vi "ElmoInterface.vi"(0 "Elmo State Cluster In":T1, 1 "Axis No.":u32, 5 "IO Signals":T2, 7 "Enable":bool, 9 "Clear faults":bool, 11 "Home":bool) -> (4 "Elmo State Cluster Out":T1, 6 "State String":string, 15 "Control word":u16)   [LabVIEW 2018]
uses:
  Clusters/IOSignals.ctl
  Clusters/ElmoState.ctl
  Clusters/SimulationConstants.ctl
  <vilib>/functionblocks/Edge Detection/Edge Detect/Edge Detect.vi
  <vilib>/functionblocks/FB Core/FB Core.xnode
  <vilib>/functionblocks/NI_FunctionBlock Libraries.lvlib
panel:
  out "Warning (Bit7)":bool
  out "Switch on disabled (Bit6)":bool
  out "Fault (Bit3)":bool
  out "Operation Enabled (Bit2)":bool
  out "Switched On (Bit1)":bool
  out "Ready to Switch On (Bit0)":bool
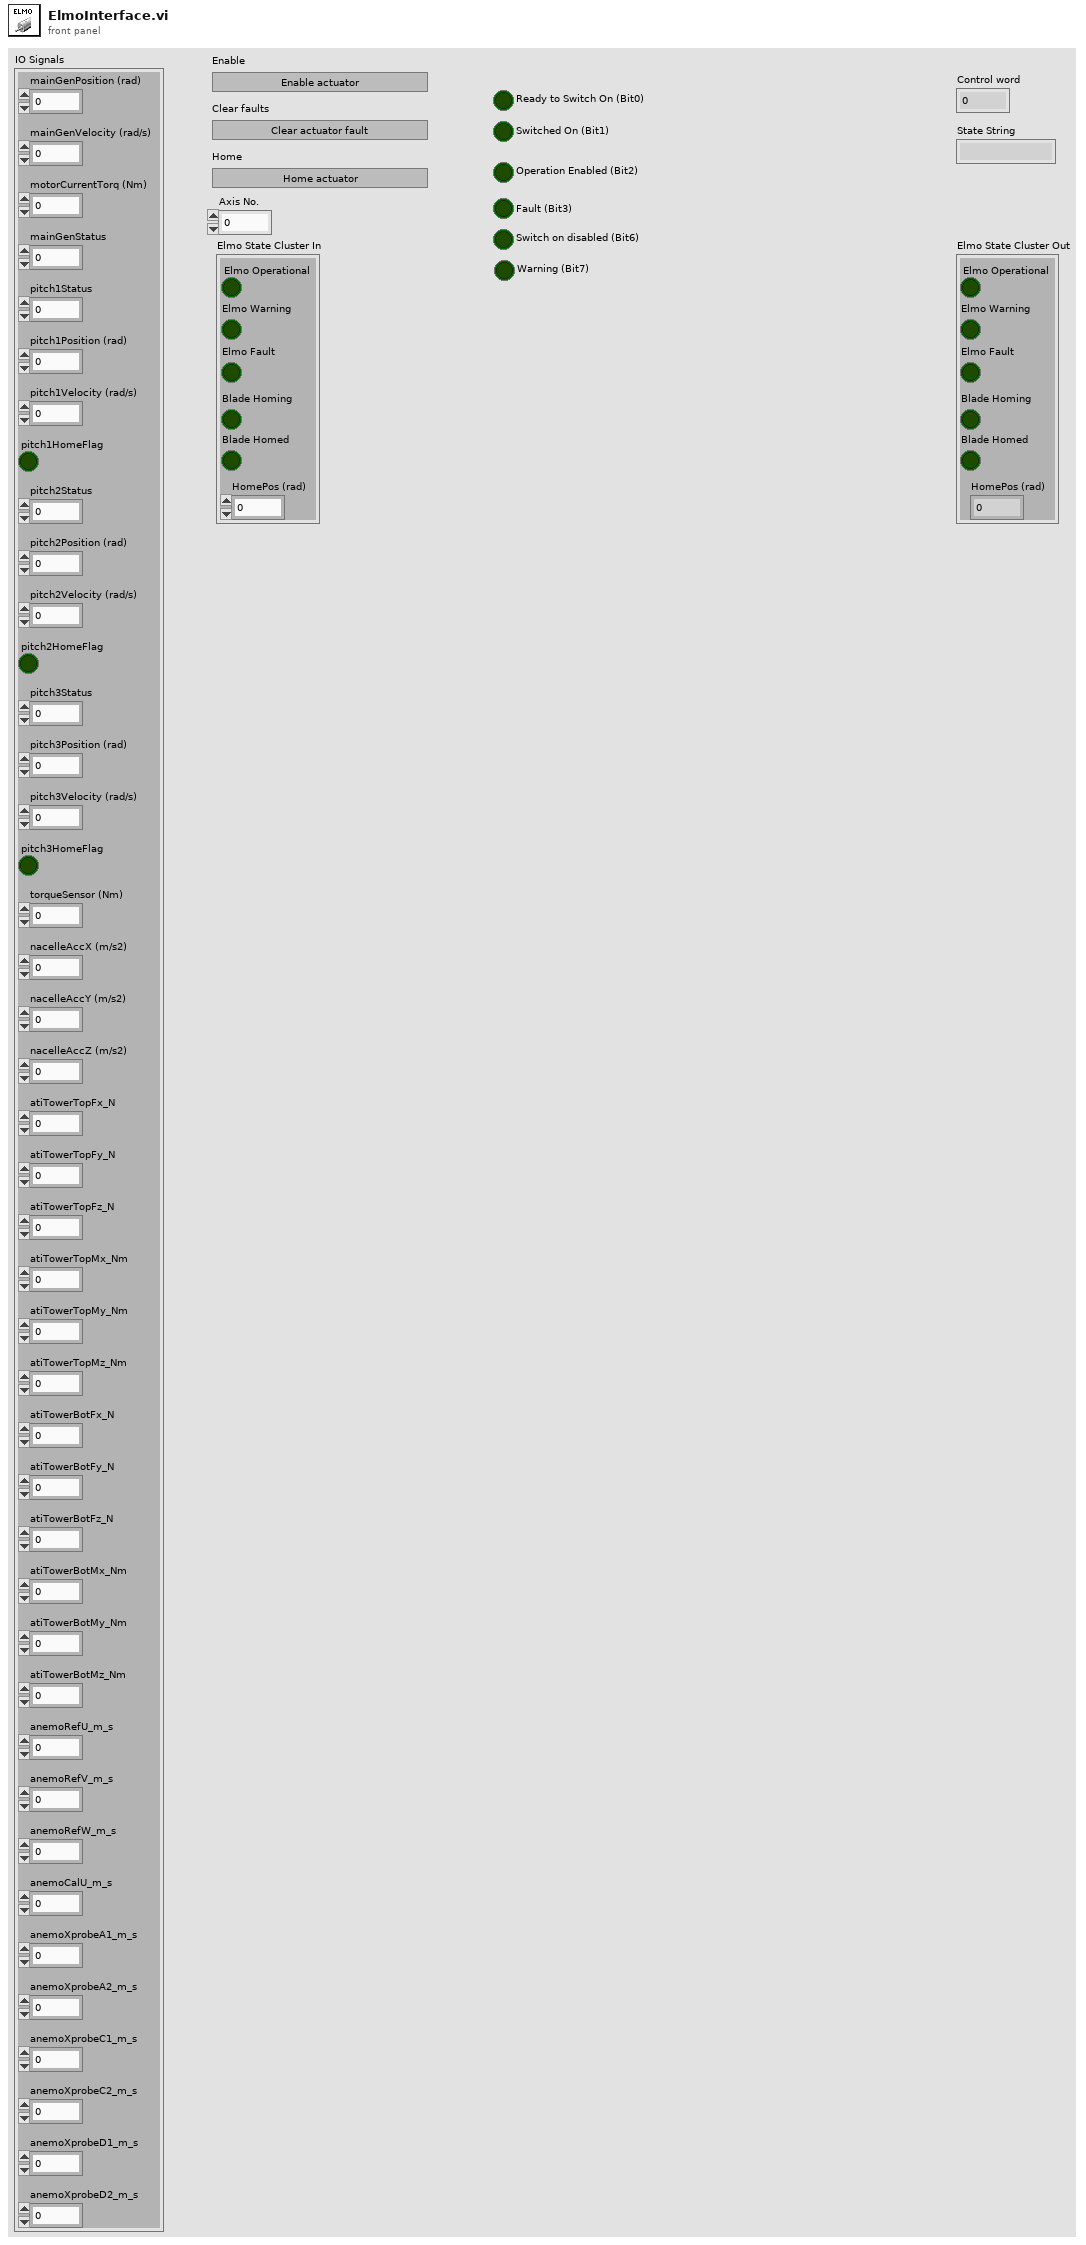
[diagram p1: front panel]
types:
  T1 = typedef "ElmoState.ctl" = cluster{"Elmo Operational":bool, "Elmo Warning":bool, "Elmo Fault":bool, "Blade Homed":bool, "Blade Homing":bool, "HomePos (rad)":dbl}
  T2 = typedef "IOSignals.ctl" = cluster{"mainGenPosition (rad)":dbl, "mainGenVelocity (rad/s)":dbl, "motorCurrentTorq (Nm)":dbl, "mainGenStatus":u16, "pitch1Status":u16, "pitch1Position (rad)":dbl, "pitch1Velocity (rad/s)":dbl, "pitch1HomeFlag":bool, "pitch2Status":u16, "pitch2Position (rad)":dbl, "pitch2Velocity (rad/s)":dbl, "pitch2HomeFlag":bool, "pitch3Status":u16, "pitch3Position (rad)":dbl, "pitch3Velocity (rad/s)":dbl, "pitch3HomeFlag":bool, "torqueSensor (Nm)":dbl, "nacelleAccX (m/s2)":dbl, "nacelleAccY (m/s2)":dbl, "nacelleAccZ (m/s2)":dbl, "atiTowerTopFx_N":dbl, "atiTowerTopFy_N":dbl, "atiTowerTopFz_N":dbl, "atiTowerTopMx_Nm":dbl, "atiTowerTopMy_Nm":dbl, "atiTowerTopMz_Nm":dbl, "atiTowerBotFx_N":dbl, "atiTowerBotFy_N":dbl, "atiTowerBotFz_N":dbl, "atiTowerBotMx_Nm":dbl, "atiTowerBotMy_Nm":dbl, "atiTowerBotMz_Nm":dbl, "anemoRefU_m_s":dbl, "anemoRefV_m_s":dbl, "anemoRefW_m_s":dbl, "anemoCalU_m_s":dbl, "anemoXprobeA1_m_s":dbl, "anemoXprobeA2_m_s":dbl, "anemoXprobeC1_m_s":dbl, "anemoXprobeC2_m_s":dbl, "anemoXprobeD1_m_s":dbl, "anemoXprobeD2_m_s":dbl}
  T3 = typedef "SimulationConstants.ctl" = cluster{"nGear":dbl, "rotorRadius":sgl, "numBlades":i32, "scaleFactor":dbl, "roscoInitMinSpeed_rad_s":dbl, "roscoInitMinTorqueFS_Nm":dbl, "beckhoff16bit":dbl, "beckhoff24BitExt":i32, "BX824Bit":i32, "rotorTorqueScale_Nm_V":dbl, "rotorTorqueOfst_Nm":dbl, "rangeEL3104V":dbl, "nacelleAccELM3604V":dbl, "nacelleAccScaleX_m_s2_V":dbl, "nacelleAccOfstX_m_s2":dbl, "nacelleAccScaleY_m_s2_V":dbl, "nacelleAccOfstY_m_s2":dbl, "nacelleAccScaleZ_m_s2_V":dbl, "nacelleAccOfstZ_m_s2":dbl, "cyberGearRatio":dbl, "cyberLinesPerRev":dbl, "cyberRatedTorque":dbl, "towerTopForceScale":dbl, "towerTopTorqueScale":dbl, "towerBotForceScale":dbl, "towerBotTorqueScale":dbl, "plcSetpointScaling_norm2VFD":dbl, "towerBotScaleMy_Nm_V":dbl, "towerBotOfstMy_Nm":dbl, "towerTopScaleXaxis_N_V":dbl, "towerTopOfstXaxis_N":dbl, "towerTopScaleYaxis_N_V":dbl, "towerTopOfstYaxis_N":dbl, "pitchFlagOffset_deg":dbl, "anemWindSpeedScaleU_m_s_m_s":dbl, "anemWindSpeedOfstU_m_s":dbl, "anemWindSpeedScaleV_m_s_m_s":dbl, "anemWindSpeedOfstV_m_s":dbl, "anemWindSpeedScaleW_m_s_m_s":dbl, "anemWindSpeedOfstW_m_s":dbl, "anemWindSpeedScaleTSI1_m_s_V":dbl, "anemWindSpeedOfstTSI1_m_s":dbl, "anemWindSpeedScaleTSI3_m_s_V":dbl, "anemWindSpeedOfstTSI3_m_s":dbl, "anemWindSpeedScaleXProbeA1C0":dbl, "anemWindSpeedScaleXProbeA1C1":dbl, "anemWindSpeedScaleXProbeA1C2":dbl, "anemWindSpeedScaleXProbeA1C3":dbl, "anemWindSpeedScaleXProbeA1C4":dbl, "anemWindSpeedOfstXProbeA1_m_s":dbl, "anemWindSpeedScaleXProbeA2C0":dbl, "anemWindSpeedScaleXProbeA2C1":dbl, "anemWindSpeedScaleXProbeA2C2":dbl, "anemWindSpeedScaleXProbeA2C3":dbl, "anemWindSpeedScaleXProbeA2C4":dbl, "anemWindSpeedOfstXProbeA2_m_s":dbl, "anemWindSpeedScaleXProbeC1C0":dbl, "anemWindSpeedScaleXProbeC1C1":dbl, "anemWindSpeedScaleXProbeC1C2":dbl, "anemWindSpeedScaleXProbeC1C3":dbl, "anemWindSpeedScaleXProbeC1C4":dbl, "anemWindSpeedOfstXProbeC1_m_s":dbl, "anemWindSpeedScaleXProbeC2C0":dbl, "anemWindSpeedScaleXProbeC2C1":dbl, "anemWindSpeedScaleXProbeC2C2":dbl, "anemWindSpeedScaleXProbeC2C3":dbl, "anemWindSpeedScaleXProbeC2C4":dbl, "anemWindSpeedOfstXProbeC2_m_s":dbl, "anemWindSpeedScaleXProbeD1C0":dbl, "anemWindSpeedScaleXProbeD1C1":dbl, "anemWindSpeedScaleXProbeD1C2":dbl, "anemWindSpeedScaleXProbeD1C3":dbl, "anemWindSpeedScaleXProbeD1C4":dbl, "anemWindSpeedOfstXProbeD1_m_s":dbl, "anemWindSpeedScaleXProbeD2C0":dbl, "anemWindSpeedScaleXProbeD2C1":dbl, "anemWindSpeedScaleXProbeD2C2":dbl, "anemWindSpeedScaleXProbeD2C3":dbl, "anemWindSpeedScaleXProbeD2C4":dbl, "anemWindSpeedOfstXProbeD2_m_s":dbl, "anemWindSpeedOfstHw3_m_s":dbl, "anemWindSpeedScaleHw3_m_s_V":dbl, "probeAOfstX_mm":dbl, "probeAOfstY_mm":dbl, "probeAOfstZ_mm":dbl, "probeTSIOfstX_mm":dbl, "probeTSIOfstY_mm":dbl, "probeTSIOfstZ_mm":dbl, "probeBOfstX_mm":dbl, "probeBOfstY_mm":dbl, "probeBOfstZ_mm":dbl}
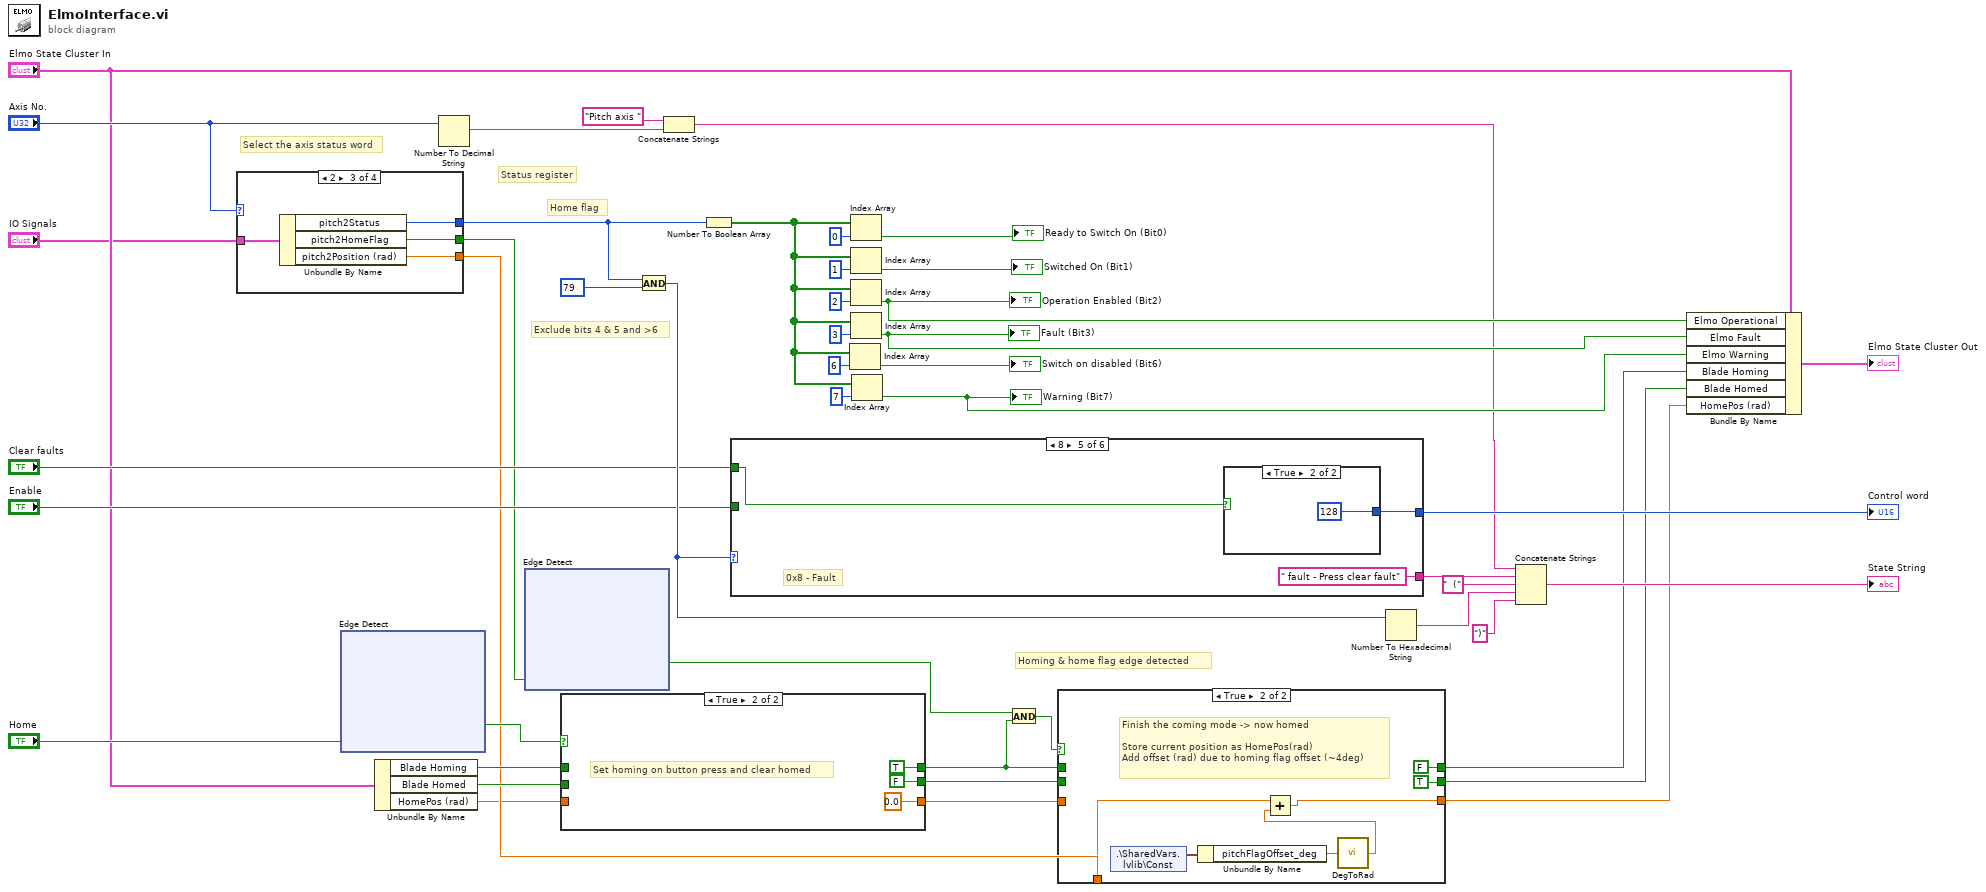
[diagram p0: block diagram]
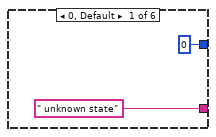
[diagram p4: hidden frame]
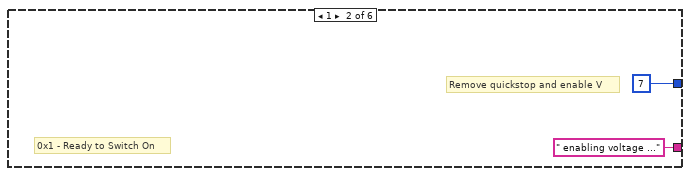
[diagram p5: hidden frame]
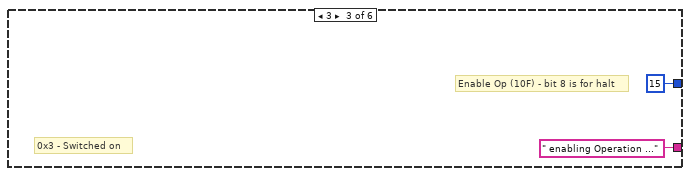
[diagram p6: hidden frame]
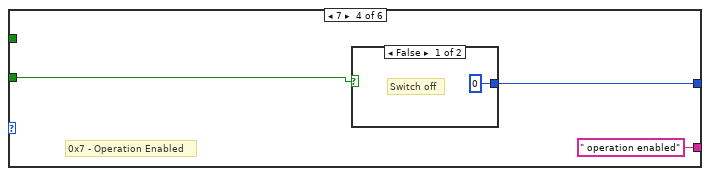
[diagram p7: hidden frame]
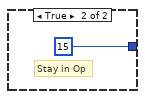
[diagram p8: hidden frame]
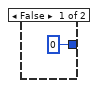
[diagram p9: hidden frame]
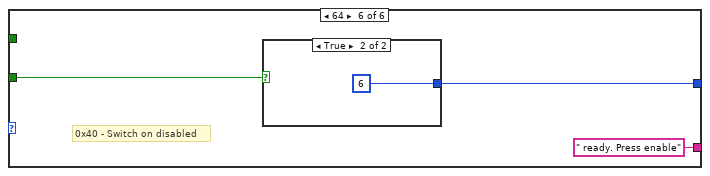
[diagram p10: hidden frame]
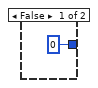
[diagram p11: hidden frame]
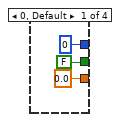
[diagram p12: hidden frame]
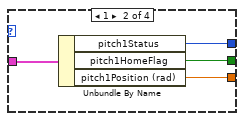
[diagram p13: hidden frame]
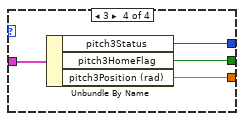
[diagram p14: hidden frame]
diagram:
  # "Homing & home flag edge detected"
  # "Home flag"
  # "Status register"
  # "Select the axis status word"
  # "Exclude bits 4 & 5 and >6"
  n1 = case shown="2" "Axis No." {
    tunnel: [u16 0 ("pitch3Status") w53 w56 w60] -> w32
    tunnel: "IO Signals" -> [_ w52 w57 w61]
    tunnel: [FALSE ("pitch3HomeFlag") w51 w55 w59] -> w6
    tunnel: [0.0 ("pitch3Position (rad)") w50 w54 w58] -> w4
    frame 0, Default {
    }
    frame 1 {
      n2 = Unbundle By Name(w52) -> ("pitch1Status"=w53:u16, "pitch1HomeFlag"=w51:bool, "pitch1Position (rad)"=w50:dbl)
    }
    frame 2 {
      n3 = Unbundle By Name(w57) -> ("pitch2Status"=w56:u16, "pitch2HomeFlag"=w55:bool, "pitch2Position (rad)"=w54:dbl)
    }
    frame 3 {
      n4 = Unbundle By Name(w61) -> ("pitch3Status"=w60:u16, "pitch3HomeFlag"=w59:bool, "pitch3Position (rad)"=w58:dbl)
    }
  }
  n5 = xnode "Edge Detect"("input 1"="Home") -> ("output"=w15:bool)  [unwired: 2 in, 1 out]
  n6 = Unbundle By Name("Elmo State Cluster In") -> ("Blade Homing"=w14:bool, "Blade Homed"=w12:bool, "HomePos (rad)"=w3:dbl)
  n7 = Number To Decimal String(number="Axis No.") -> (decimal integer string=w20:string)  [unwired: 1 in]
  n8 = xnode "Edge Detect"("input 1"=w6) -> ("output"=w5:bool)  [unwired: 2 in, 1 out]
  n9 = case shown="True" w15 {
    tunnel: w14 -> [w64 _]
    tunnel: [w64 TRUE ("Blade Homing")] -> w10
    tunnel: w12 -> [w63 _]
    tunnel: [w63 FALSE ("Blade Homed")] -> w9
    tunnel: w3 -> [w62 _]
    tunnel: [w62 0.0 ("HomePos (rad)")] -> w2
    frame False {
      # "Stay in present mode"
    }
    frame True {
      # "Set homing on button press and clear homed"
    }
  }
  n10 = And(x=w32, y=u16 79) -> (x .and. y?=w30:u16)
  n11 = Concatenate Strings("Pitch axis " ("string"), w20) -> (w19:string)
  n12 = Number To Boolean Array(number=w32) -> (Boolean array=w37:bool[])
  n13 = case shown="8" w30 {
    tunnel: [" unknown state" ("AccelNet State") " enabling voltage ..." ("AccelNet State") " enabling Operation ..." ("AccelNet State") " operation enabled" ("AccelNet State") " fault - Press clear fault" ("AccelNet State") " ready. Press enable" ("AccelNet State")] -> w36
    tunnel: "Enable" -> [_ _ _ w74 _ w85]
    tunnel: [u16 0 ("Control word") u16 7 ("Control word") u16 15 ("Control word") w75 w79 w84] -> w27
    tunnel: "Clear faults" -> [_ _ _ _ w80 _]
    frame 0, Default {
    }
    frame 1 {
      # "Remove quickstop and enable V"
      # "0x1 - Ready to Switch On"
    }
    frame 3 {
      # "Enable Op (10F) - bit 8 is for halt"
      # "0x3 - Switched on"
    }
    frame 7 {
      # "0x7 - Operation Enabled"
      n14 = case shown="False" w74 {
        tunnel: [u16 0 ("Control word") u16 15 ("Control word")] -> w75
        frame False {
          # "Switch off"
        }
        frame True {
          # "Stay in Op"
        }
      }
    }
    frame 8 {
      # "0x8 - Fault"
      n15 = case shown="True" w80 {
        tunnel: [u16 0 ("Control word") u16 128 ("Control word")] -> w79
        frame False {
        }
        frame True {
        }
      }
    }
    frame 64 {
      # "0x40 - Switch on disabled"
      n16 = case shown="True" w85 {
        tunnel: [u16 0 ("Control word") u16 6 ("Control word")] -> w84
        frame False {
        }
        frame True {
        }
      }
    }
  }
  "Control word" <- w27
  n17 = Index Array(array=w37, index=6) -> (element=→"Switch on disabled (Bit6)":bool)
  n18 = Index Array(array=w37, index=0) -> (element=→"Ready to Switch On (Bit0)":bool)
  n19 = Index Array(array=w37, index=1) -> (element=→"Switched On (Bit1)":bool)
  n20 = Index Array(array=w37, index=2) -> (element=w26:bool)
  "Operation Enabled (Bit2)" <- w26
  n21 = Index Array(array=w37, index=3) -> (element=w29:bool)
  "Fault (Bit3)" <- w29
  n22 = Index Array(array=w37, index=7) -> (element=w28:bool)
  "Warning (Bit7)" <- w28
  n23 = And(x=w5, y=w10) -> (x .and. y?=w11:bool)
  n24 = case shown="True" w11 {
    tunnel: w10 -> [w91 _]
    tunnel: w9 -> [w90 _]
    tunnel: [w91 FALSE ("Blade Homing")] -> w8
    tunnel: [w90 TRUE ("Blade Homed")] -> w7
    tunnel: w4 -> [_ w95]
    tunnel: w2 -> [w89 _]
    tunnel: [w89 w96] -> w1
    frame False {
      # "Stay in current mode"
    }
    frame True {
      # "Finish the coming mode -> now homed\n\nStore current position as HomePos(rad)\nAdd offset (rad) due to homing flag offset (~4deg)"
      n25 = shared-variable ".\\SharedVars.lvlib\\Const"() -> (w94:T3)  [unwired: 1 in, 1 out]
      n26 = Unbundle By Name(w94) -> ("pitchFlagOffset_deg"=w93:dbl)
      n27 = call "DegToRad.vi"("deg"=w93) -> ("rad"=w92:dbl)
      n28 = Add(x=w95, y=w92) -> (x+y=w96:dbl)
    }
  }
  n29 = Number To Hexadecimal String(2:w30) -> (0:w33:string)  [unwired: 1 in]
  n30 = Concatenate Strings(w19, w36, "  (" ("string"), w33, ")" ("string")) -> (→"State String":string)
  n31 = Bundle By Name(cluster="Elmo State Cluster In", "Elmo Operational"=w26, "Elmo Fault"=w29, "Elmo Warning"=w28, "Blade Homing"=w8, "Blade Homed"=w7, "HomePos (rad)"=w1) -> (→"Elmo State Cluster Out":T1)
